vi "PQdescribePrepared.vi"(8 "error in (no error)":errorcluster, 10 "stmtName":string, 11 "conn":u32) -> (0 "error out":errorcluster, 2 "res":u32, 3 "conn_out":u32)   [LabVIEW 2019, in "libpqlv.lvlib"]
doc: "Submits a request to obtain information about the specified prepared statement, and waits for completion. PGresult *PQdescribePrepared(PGconn *conn, const char *stmtName);\nhttp://www.postgresql.org/docs/8.3/static/libpq-exec.html"
uses:
  libpqlv.lvlib
  libpq.dll
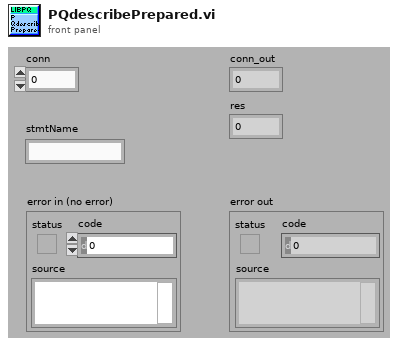
[diagram p1: front panel]
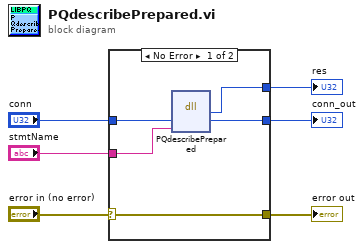
[diagram p0: block diagram]
diagram:
  n1 = case shown="No Error" "error in (no error)" {
    selector: "error in (no error)" -> [w11 w13]
    tunnel: [w11 w13] -> w5
    tunnel: [w10 _] -> w4
    tunnel: [w9 w12] -> w2
    tunnel: "stmtName" -> [w8 _]
    tunnel: "conn" -> [w7 w12]
    frame No Error {
      n2 = dll-call lib="libpq.*" fn="PQdescribePrepared"("conn"=w7, "stmtName"=w8) -> ("PQdescribePrepared"=w10:u32, "conn"=w9:u32)  [unwired: 4 in, 2 out]
    }
    frame Error {
    }
  }
  "res" <- w4
  "error out" <- w5
  "conn_out" <- w2
